vi "Open_All_Relays_except_PNEU_P.2.2.vi"(1 "Delay Time (s)":dbl=0.1, 3 "error in":errorcluster) -> (10 "error out":errorcluster)   [LabVIEW 2015]
uses:
  <vilib>/DAQmx/write.llb/DAQmx Write (Digital 1D Bool 1Chan 1Samp).vi
  <vilib>/DAQmx/create/channels.llb/DAQmx Create Channel (DO-Digital Output).vi
  <vilib>/DAQmx/miscellaneous.llb/DAQmx Fill In Error Info.vi
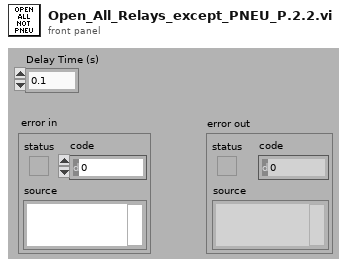
[diagram p1: front panel]
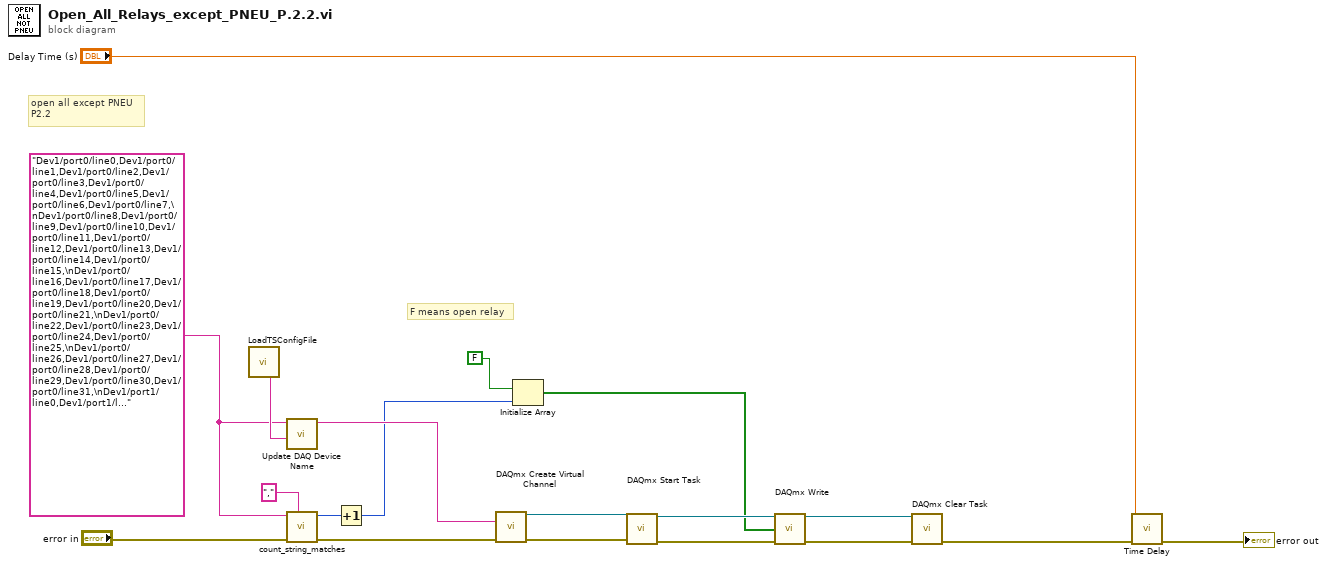
[diagram p0: block diagram]
diagram:
  w3 = "Dev1/port0/line0,Dev1/port0/line1,Dev1/port0/line2,Dev1/port0/line3,Dev1/port0/line4,Dev1/port0/line5,Dev1/port0/line6,Dev1/port0/line7,\nDev1/port0/line8,Dev1/port0/line9,Dev1/port0/line10,Dev1/port0/line11,Dev1/port0/line12,Dev1/port0/line13,Dev1/port0/line14,Dev1/port0/line15,\nDev1/port0/line16,Dev1/port0/line17,Dev1/port0/line18,Dev1/port0/line19,Dev1/port0/line20,Dev1/port0/line21,\nDev1/port0/line22,Dev1/port0/line23,Dev1/port0/line24,Dev1/port0/line25,\nDev1/port0/line26,Dev1/port0/line27,Dev1/port0/line28,Dev1/port0/line29,Dev1/port0/line30,Dev1/port0/line31,\nDev1/port1/line0,Dev1/port1/line1,Dev1/port1/line2,Dev1/port1/line3,Dev1/port1/line4,Dev1/port1/line5,Dev1/port1/line6,Dev1/port1/line7,\nDev1/port2/line0,Dev1/port2/line1,Dev1/port2/line3,Dev1/port2/line4,Dev1/port2/line5,Dev1/port2/line6,Dev1/port2/line7\n"
  # "open all except PNEU\nP2.2"
  # "F means open relay"
  n1 = call "LoadTSConfigFile.vi"() -> ("DAQDevice"=w5:string)  [unwired: 5 in, 10 out]
  n2 = call "Update DAQ Device Name.vi"("Device Name"=w5, "Lines in (String)"=w3) -> ("Lines out (DAQmx Physical Channels)"=w11:tag)  [unwired: 9 in]
  n3 = call "count_string_matches.vi"("String"=w3, "error in (no error)"="error in", "String to Match"=",") -> ("Number of matches"=w19:i32, "error out"=w10:errorcluster)  [unwired: 6 in]
  n4 = Increment(x=w19) -> (x+1=w7:i32)
  n5 = call-poly <vilib>:"DAQmx Create Virtual Channel.vi"("lines"=w11, "error in"=w10) -> ("task out"=w16:refnum<k21>, "error out"=w17:errorcluster)  [unwired: 12 in]
  n6 = Initialize Array(FALSE ("Boolean"), w7) -> (w6:bool[])
  n7 = call <vilib>:"DAQmx Start Task.vi"("task/channels in"=w16, "error in"=w17) -> ("task out"=w15:refnum<k21>, "error out"=w14:errorcluster)  [unwired: 12 in]
  n8 = call-poly <vilib>:"DAQmx Write.vi"("task/channels in"=w15, "data"=w6, "error in"=w14) -> ("task out"=w13:refnum<k21>, "error out"=w12:errorcluster)  [unwired: 10 in, 1 out]
  n9 = call <vilib>:"DAQmx Clear Task.vi"("task in"=w13, "error in"=w12) -> ("error out"=w8:errorcluster)  [unwired: 13 in]
  n10 = call "Time Delay"("error in (no error)"=w8, "Delay Time (s)"="Delay Time (s)") -> ("error out"=→"error out":errorcluster)  [unwired: 9 in]
